vi "Advanced Power Measurement (DAQmx).vi"() -> ()   [LabVIEW 2024]
doc: "Demonstrates how to implement advanced power measurement on a three-phase electrical power system. This example VI measures the electrical power parameters, such as voltage and current RMS values, power and energy values, frequency amplitudes, etc, with a higher accuracy by grouping the signals into integral cycles."
uses:
  <vilib>/Utility/error.llb/DialogType.ctl
  <vilib>/DAQmx/read.llb/DAQmx Read (Analog 1D Wfm NChan NSamp).vi
  <vilib>/addons/Electrical Power/Basic/Measurement/RMS (N Channels).vi
  <vilib>/addons/Electrical Power/Basic/Measurement/RMS (1 Channel).vi
  <vilib>/Analysis/5stat.llb/RMS (DBL).vi
  <vilib>/DAQmx/create/channels.llb/DAQmx Create Channel (AI-Voltage-Basic).vi
  <vilib>/DAQmx/create/channels.llb/DAQmx Create Channel (AI-Current-Basic).vi
  <vilib>/DAQmx/configure/timing.llb/DAQmx Timing (Sample Clock).vi
  <vilib>/DAQmx/miscellaneous.llb/DAQmx Fill In Error Info.vi
  <vilib>/measure/maUtilsandCtls.llb/ma_Check Waveform Timing.vi
  <vilib>/addons/Electrical Power/Basic/Measurement/Fundamental Vector (N Channels).vi
  <vilib>/addons/Electrical Power/Basic/Measurement/Power (N Channels).vi
  <vilib>/addons/Electrical Power/Basic/Measurement/Energy (N Channels).vi
  <resource>/objmgr/daqmx.rc
  <vilib>/addons/Electrical Power/Power Measurement/NI_EP_Power Measurement.lvlib
  <vilib>/addons/Electrical Power/Basic/NI_EP_Basic.lvlib
panel:
  in  "Tab Control":T1(tab)
  in  "minimum voltage value":dbl=-300.0 format="%0.2f"
  in  "maximum voltage value":dbl=300.0 format="%0.2f"
  in  "voltage channels":tag
  in  "minimum current value":dbl=-5.0 format="%0.2f"
  in  "maximum current value":dbl=5.0 format="%0.2f"
  in  "current channels":tag
  in  "DAQmx sample rate [Hz]":dbl=50000.0 format="%0.2f"
  in  "number of samples per channel":i32=10000
  in  "frequency range [Hz]":cluster{"minimum":dbl, "maximum":dbl}={"minimum"=45.0, "maximum"=55.0}
  in  "filter for frequency measurement":T2={"enable filter? (T)"=TRUE, "passband edge frequency [Hz]"=55.0, "passband ripple [dB]"=0.1, "stopband edge frequency [Hz]"=85.0, "stopband attenuation [dB]"=60.0}
  out "Voltage Waveforms":waveform(dbl)[](graph)
  out "actual DAQmx \nsample rate  [Hz]":dbl
  out "average frequency [Hz]":dbl
  out "Current Waveforms":waveform(dbl)[](graph)
  out "voltage RMS values":dbl[](array[numeric])
  out "current RMS values":dbl[](array[numeric])
  out "phase difference [deg]":dbl[](array[numeric])
  out "minimum voltage [V]":dbl[](array[numeric])
  out "maximum voltage [V]":dbl[](array[numeric])
  out "voltage DC values":dbl[](array[numeric])
  out "voltage ARVs":dbl[](array[numeric])
  out "voltage calibrated ARVs":dbl[](array[numeric])
  out "voltage crest factor":dbl[](array[numeric])
  out "power values":T3(array[cluster])
  out "energy values":T4(array[cluster])
  in  "stop":bool
  # "Overview: Demonstrates how to implement advanced power measurement on a three-phase electrical power system.\nRequirements: NI-DAQmx, Electrical Power Toolkit Full Edition\nInstructions: 1. Connect the signals you want to perform advanced power measurement to the DAQ devices.\n                        2. Configure Settings and run this VI."
  # "DAQmx"
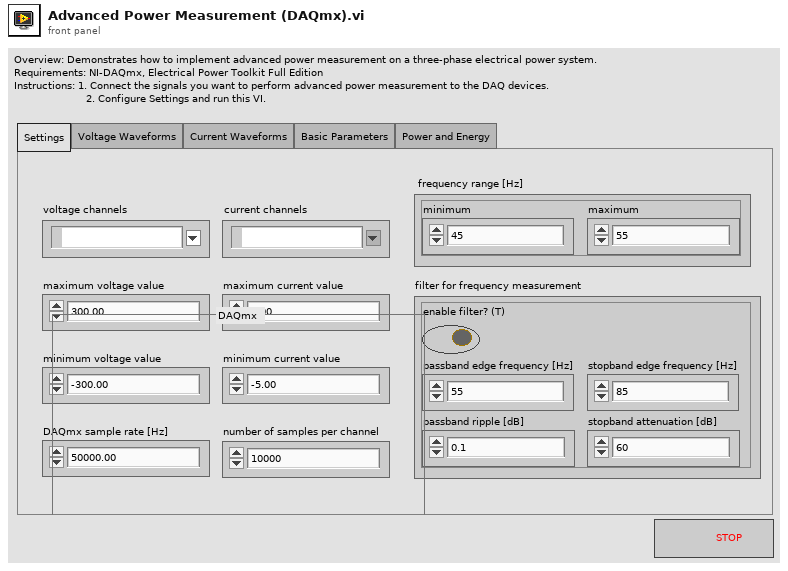
[diagram p1: front panel]
types:
  T1 = enum32{"Settings", "Voltage Waveforms", "Current Waveforms", "Basic Parameters", "Power and Energy"}
  T2 = cluster{"enable filter? (T)":bool, "passband edge frequency [Hz]":dbl, "passband ripple [dB]":dbl, "stopband edge frequency [Hz]":dbl, "stopband attenuation [dB]":dbl}
  T3 = cluster{"active power [W]":dbl, "apparent power [VA]":dbl, "reactive power [VAR]":dbl, "power factor":dbl}[]
  T4 = cluster{"active energy [Wh]":dbl, "apparent energy [VAh]":dbl, "reactive energy [VARh]":dbl}[]
  T5 = typedef "DialogType.ctl" = u16
  T6 = cluster{"zero crossing times [s]":dbl[], "zero crossings per cycle":u8}
  T7 = typedef "NI_EP_Basic.lvlib/basic_Power Value.ctl" = cluster{"active power [W]":dbl, "apparent power [VA]":dbl, "reactive power [VAR]":dbl, "power factor":dbl}
  T8 = typedef "NI_EP_Basic.lvlib/basic_Energy Value.ctl" = cluster{"active energy [Wh]":dbl, "apparent energy [VAh]":dbl, "reactive energy [VARh]":dbl}
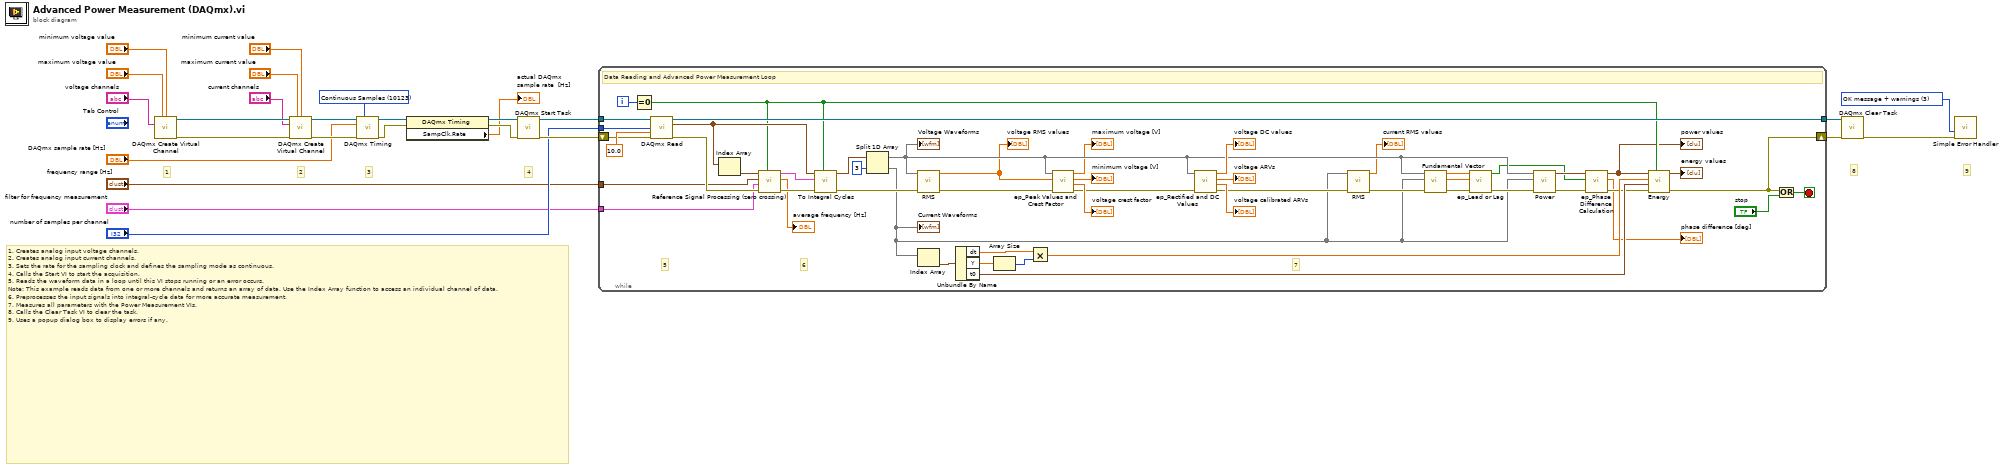
[diagram p0: block diagram]
diagram:
  w1 = 10123 items=["Finite Samples"=10178, "Continuous Samples"=10123, "Hardware Timed Single Point"=12522] ("sample mode")
  w5 = T5 3 items=["no dialog", "OK message", "continue or stop message", "OK message + warnings", "continue/stop + warnings"] ("type of dialog (OK msg:1)")
  # "1. Creates analog input voltage channels.\n2. Creates analog input current channels.\n3. Sets the rate for the sampling clock and defines the sampling mode as continuous.\n4. Calls the Start VI to start the acquisition.\n5. Reads the waveform data in a loop until this VI stops running or an error occurs.\nNote: This example reads data from one or more channels and returns an array of data. Use the Index Array function to access an individual channel of data.\n6. Preprocesses the input signals into integral-cycle data for more accurate measurement. \n7. Measures all parameters with the Power Measurement VIs.\n8. Calls the Clear Task VI to clear the task.\n9. Uses a popup dialog box to display errors if any."
  # "9"
  # "8"
  # "4"
  # "3"
  # "2"
  # "1"
  n1 = call-poly <vilib>:"DAQmx Create Virtual Channel.vi"("maximum value"="maximum voltage value", "minimum value"="minimum voltage value", "physical channels"="voltage channels") -> ("task out"=w22:refnum<k21>, "error out"=w23:errorcluster)  [unwired: 11 in]
  n2 = call-poly <vilib>:"DAQmx Create Virtual Channel.vi"("task in"=w22, "maximum value"="maximum current value", "minimum value"="minimum current value", "physical channels"="current channels", "error in"=w23) -> ("task out"=w17:refnum<k21>, "error out"=w18:errorcluster)  [unwired: 9 in]
  n3 = call-poly <vilib>:"DAQmx Timing.vi"("task/channels in"=w17, "sample mode"=w1, "rate"="DAQmx sample rate [Hz]", "error in"=w18) -> ("task out"=w10:refnum<k21>, "error out"=w15:errorcluster)  [unwired: 10 in]
  n4 = property class="DAQmx Timing"(reference=w10, error in=w15) -> (reference out=w14:refnum<k21>, error out=w13:errorcluster, "SampClk.Rate"=→"actual DAQmx \nsample rate  [Hz]":dbl)
  n5 = call <vilib>:"DAQmx Start Task.vi"("task/channels in"=w14, "error in"=w13) -> ("task out"=w12:refnum<k21>, "error out"=w11:errorcluster)  [unwired: 12 in]
  n6 = while {
    tunnel: "number of samples per channel" -> [w77]
    tunnel: w12 -> [w78]
    tunnel: [w76] -> w4
    shift-right: [w61] -> w7
    shift-left: w11 -> [w67]
    tunnel: "frequency range [Hz]" -> [w60]
    tunnel: "filter for frequency measurement" -> [w59]
    i -> [w72]
    stop <- w73 stop-if-true
    # "7"
    # "6"
    # "5"
    # "Data Reading and Advanced Power Measurement Loop"
    n7 = Equal To 0?(x=w72) -> (x = 0?=w64:bool)
    n8 = call-poly <vilib>:"DAQmx Read.vi"("task/channels in"=w78, "number of samples per channel"=w77, "timeout"=10.0, "error in"=w67) -> ("task out"=w76:refnum<k21>, "data"=w69:waveform(dbl)[], "error out"=w75:errorcluster)  [unwired: 9 in]
    n9 = Index Array(array=w69) -> (element=w68:waveform(dbl))  [unwired: 1 in]
    n10 = call <vilib>:"Reference Signal Processing (zero crossing).vi"("reset? (F)"=w64, "error in (no error)"=w75, "filter for frequency measurement"=w59, "frequency range [Hz]"=w60, "reference signal"=w68) -> ("error out"=w74:errorcluster, "average frequency [Hz]"=→"average frequency [Hz]":dbl, "zero crossing information"=w70:T6)  [unwired: 3 in, 1 out]
    n11 = call <vilib>:"To Integral Cycles.vi"("reset? (F)"=w64, "error in (no error)"=w74, "trigger information"=w70, "data in"=w69) -> ("error out"=w48:errorcluster, "integral-cycle data"=w66:waveform(dbl)[])  [unwired: 6 in]
    n12 = Split 1D Array(array=w66, index=3) -> (first subarray=w53:waveform(dbl)[], second subarray=w40:waveform(dbl)[])
    "Voltage Waveforms" <- w53
    "Current Waveforms" <- w40
    n13 = call-poly <vilib>:"RMS.vi"("error in (no error)"=w48, "waveforms"=w53) -> ("error out"=w54:errorcluster, "RMS values"=w52:dbl[])  [unwired: 8 in]
    "voltage RMS values" <- w52
    n14 = Index Array(array=w40) -> (element=w39:waveform(dbl))  [unwired: 1 in]
    n15 = Unbundle By Name(w39) -> ("dt"=w37:dbl, "Y"=w38:dbl[], "t0"=w35:timestamp)
    n16 = Array Size(array=w38) -> (size(s)=w36:i32)
    n17 = Multiply(x=w37, y=w36) -> (x*y=w34:dbl)
    n18 = call "ep_Peak Values and Crest Factor.vi"("error in (no error)"=w54, "RMS"=w52, "data"=w53) -> ("error out"=w47:errorcluster, "crest factor"=→"voltage crest factor":dbl[], "- peak values"=→"minimum voltage [V]":dbl[], "+peak values"=→"maximum voltage [V]":dbl[])  [unwired: 5 in]
    n19 = call "ep_Rectified and DC Values.vi"("error in (no error)"=w47, "data"=w53) -> ("error out"=w44:errorcluster, "calibrated ARVs"=→"voltage calibrated ARVs":dbl[], "ARVs"=→"voltage ARVs":dbl[], "DC values"=→"voltage DC values":dbl[])  [unwired: 6 in]
    n20 = call-poly <vilib>:"RMS.vi"("error in (no error)"=w44, "waveforms"=w40) -> ("error out"=w43:errorcluster, "RMS values"=→"current RMS values":dbl[])  [unwired: 8 in]
    n21 = call-poly <vilib>:"Fundamental Vector.vi"("error in (no error)"=w43, "current waveforms"=w40, "voltage waveforms"=w53) -> ("error out"=w45:errorcluster, "current fundamental vectors"=w46:cdb[], "voltage fundamental vectors"=w28:cdb[])  [unwired: 5 in, 1 out]
    n22 = call "ep_Lead or Lag.vi"("error in (no error)"=w45, "current fundamental vectors"=w46, "voltage fundamental vectors"=w28) -> ("error out"=w41:errorcluster, "lead/lag ? (T)"=w27:bool[])  [unwired: 7 in]
    n23 = call-poly <vilib>:"Power.vi"("error in (no error)"=w41, "current waveforms"=w40, "voltage waveforms"=w53) -> ("error out"=w33:errorcluster, "power values"=w31:T7[])  [unwired: 7 in]
    n24 = call "ep_Phase Difference Calculation.vi"("error in (no error)"=w33, "lead/lag ? (T)"=w27, "power values in"=w31) -> ("error out"=w32:errorcluster, "phase difference [deg]"=→"phase difference [deg]":dbl[], "power values out"=w30:T7[])  [unwired: 6 in]
    "power values" <- w30
    n25 = call-poly <vilib>:"Energy.vi"("reset? (F)"=w64, "error in (no error)"=w32, "start timestamp"=w35, "interval length [s]"=w34, "power values"=w30) -> ("error out"=w61:errorcluster, "energy values"=→"energy values":T8[])  [unwired: 4 in, 1 out]
    n26 = Or(x=w61, y="stop") -> (x .or. y?=w73:bool)
  }
  n27 = call <vilib>:"DAQmx Clear Task.vi"("task in"=w4, "error in"=w7) -> ("error out"=w6:errorcluster)  [unwired: 13 in]
  n28 = call <vilib>:"Simple Error Handler.vi"("type of dialog (OK msg:1)"=w5, "error in (no error)"=w6) -> ()  [unwired: 3 in, 5 out]
